vi "NF LI56xx u_err_setSource.vi"(11 "error in (no error)":errorcluster) -> (3 "error out":errorcluster)   [LabVIEW 2019]
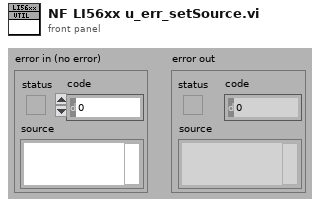
[diagram p1: front panel]
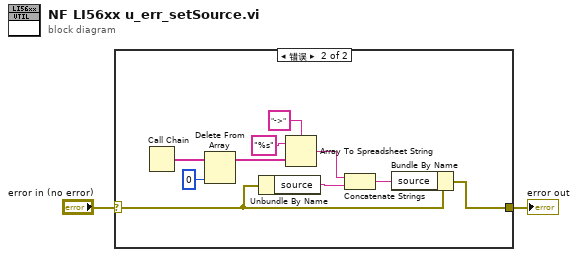
[diagram p0: block diagram]
diagram:
  n1 = case shown="错误" "error in (no error)" {
    selector: "error in (no error)" -> [w3 w12]
    tunnel: [w3 w13] -> w2
    frame No Error {
    }
    frame Error {
      n2 = Call Chain() -> (call chain=w6:string[])
      n3 = Delete From Array(array=w6, index=0 ("Žw•W")) -> (array with subset deleted=w5:string[])  [unwired: 1 in, 1 out]
      n4 = Unbundle By Name(w12) -> ("source"=w7:string)
      n5 = Array To Spreadsheet String(delimiter (Tab)="->" ("デリメタ(タブ)"), array=w5, 3:"%s" ("Œ`Ž®•¶Žš—ñ")) -> (spreadsheet string=w9:string)
      n6 = Concatenate Strings(w9, w7) -> (w8:string)
      n7 = Bundle By Name(cluster=w12, "source"=w8) -> (w13:errorcluster)
    }
  }
  "error out" <- w2
